vi "FPGA Main.vi"   [LabVIEW 2020]
uses:
  <vilib>/rvi/Emulation/niFpgaGetClockAttributes.vi
  <vilib>/rvi/Emulation/niFpgaSctlEmulationGetInTimedLoop.vi
  <vilib>/rvi/Emulation/niFpgaEmulationReportErrorSimple.vi
  <vilib>/rvi/Emulation/niFpgaCriticalErrorInLSC.vi
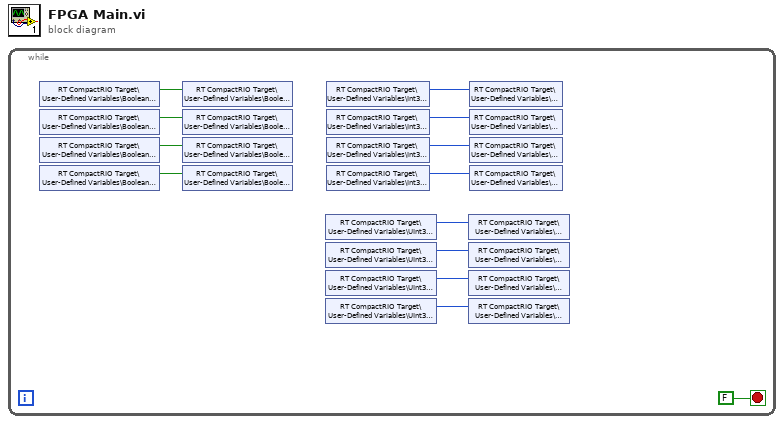
[diagram p0: block diagram]
diagram:
  n1 = while {
    stop <- FALSE stop-if-true
    n2 = shared-variable "RT CompactRIO Target\\User-Defined Variables\\Boolean Out 1"() -> (w12:bool)  [unwired: 1 in, 1 out]
    n3 = shared-variable "RT CompactRIO Target\\User-Defined Variables\\Boolean Out 2"() -> (w11:bool)  [unwired: 1 in, 1 out]
    n4 = shared-variable "RT CompactRIO Target\\User-Defined Variables\\Boolean Out 3"() -> (w10:bool)  [unwired: 1 in, 1 out]
    n5 = shared-variable "RT CompactRIO Target\\User-Defined Variables\\Boolean Out 4"() -> (w9:bool)  [unwired: 1 in, 1 out]
    n6 = shared-variable "RT CompactRIO Target\\User-Defined Variables\\Boolean In 1"(w12) -> ()  [unwired: 1 in, 1 out]
    n7 = shared-variable "RT CompactRIO Target\\User-Defined Variables\\Boolean In 2"(w11) -> ()  [unwired: 1 in, 1 out]
    n8 = shared-variable "RT CompactRIO Target\\User-Defined Variables\\Boolean In 3"(w10) -> ()  [unwired: 1 in, 1 out]
    n9 = shared-variable "RT CompactRIO Target\\User-Defined Variables\\Boolean In 4"(w9) -> ()  [unwired: 1 in, 1 out]
    n10 = shared-variable "RT CompactRIO Target\\User-Defined Variables\\UInt32 Out 1"() -> (w4:u32)  [unwired: 1 in, 1 out]
    n11 = shared-variable "RT CompactRIO Target\\User-Defined Variables\\UInt32 Out 2"() -> (w3:u32)  [unwired: 1 in, 1 out]
    n12 = shared-variable "RT CompactRIO Target\\User-Defined Variables\\UInt32 Out 3"() -> (w2:u32)  [unwired: 1 in, 1 out]
    n13 = shared-variable "RT CompactRIO Target\\User-Defined Variables\\UInt32 Out 4"() -> (w1:u32)  [unwired: 1 in, 1 out]
    n14 = shared-variable "RT CompactRIO Target\\User-Defined Variables\\Int32 Out 1"() -> (w5:i32)  [unwired: 1 in, 1 out]
    n15 = shared-variable "RT CompactRIO Target\\User-Defined Variables\\Int32 Out 2"() -> (w6:i32)  [unwired: 1 in, 1 out]
    n16 = shared-variable "RT CompactRIO Target\\User-Defined Variables\\Int32 Out 3"() -> (w7:i32)  [unwired: 1 in, 1 out]
    n17 = shared-variable "RT CompactRIO Target\\User-Defined Variables\\Int32 Out 4"() -> (w8:i32)  [unwired: 1 in, 1 out]
    n18 = shared-variable "RT CompactRIO Target\\User-Defined Variables\\UInt32 In 1"(w4) -> ()  [unwired: 1 in, 1 out]
    n19 = shared-variable "RT CompactRIO Target\\User-Defined Variables\\UInt32 In 2"(w3) -> ()  [unwired: 1 in, 1 out]
    n20 = shared-variable "RT CompactRIO Target\\User-Defined Variables\\UInt32 In 3"(w2) -> ()  [unwired: 1 in, 1 out]
    n21 = shared-variable "RT CompactRIO Target\\User-Defined Variables\\UInt32 In 4"(w1) -> ()  [unwired: 1 in, 1 out]
    n22 = shared-variable "RT CompactRIO Target\\User-Defined Variables\\Int32 In 1"(w5) -> ()  [unwired: 1 in, 1 out]
    n23 = shared-variable "RT CompactRIO Target\\User-Defined Variables\\Int32 In 2"(w6) -> ()  [unwired: 1 in, 1 out]
    n24 = shared-variable "RT CompactRIO Target\\User-Defined Variables\\Int32 In 3"(w7) -> ()  [unwired: 1 in, 1 out]
    n25 = shared-variable "RT CompactRIO Target\\User-Defined Variables\\Int32 In 4"(w8) -> ()  [unwired: 1 in, 1 out]
  }
